vi "iWorx Respiration SubVI.vi"(7 "Waveform Chart":refnum<vi>, 9 "low Threshold":dbl, 10 "high Threshold":dbl) -> (0 "Breath Time History":timestamp[](array[timestamp]), 1 "Instantaneous Breath Rate":dbl format="%.2f", 2 "Avg Breaths per Minute":dbl format="%.2f", 3 "Breath Count":u32)   [LabVIEW 2014]
doc: "This subVI is designed to work with the iWorx Respiration Sensor. It counts the number of times the signal crosses two seperate threasholds. The two threshold method allows it to more accuratly count breaths without noise.s"
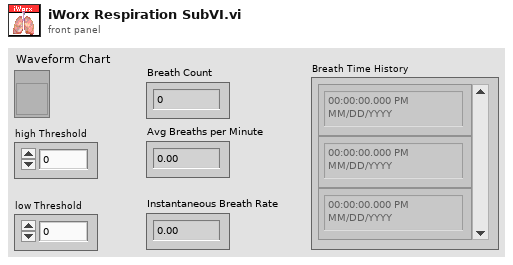
[diagram p1: front panel]
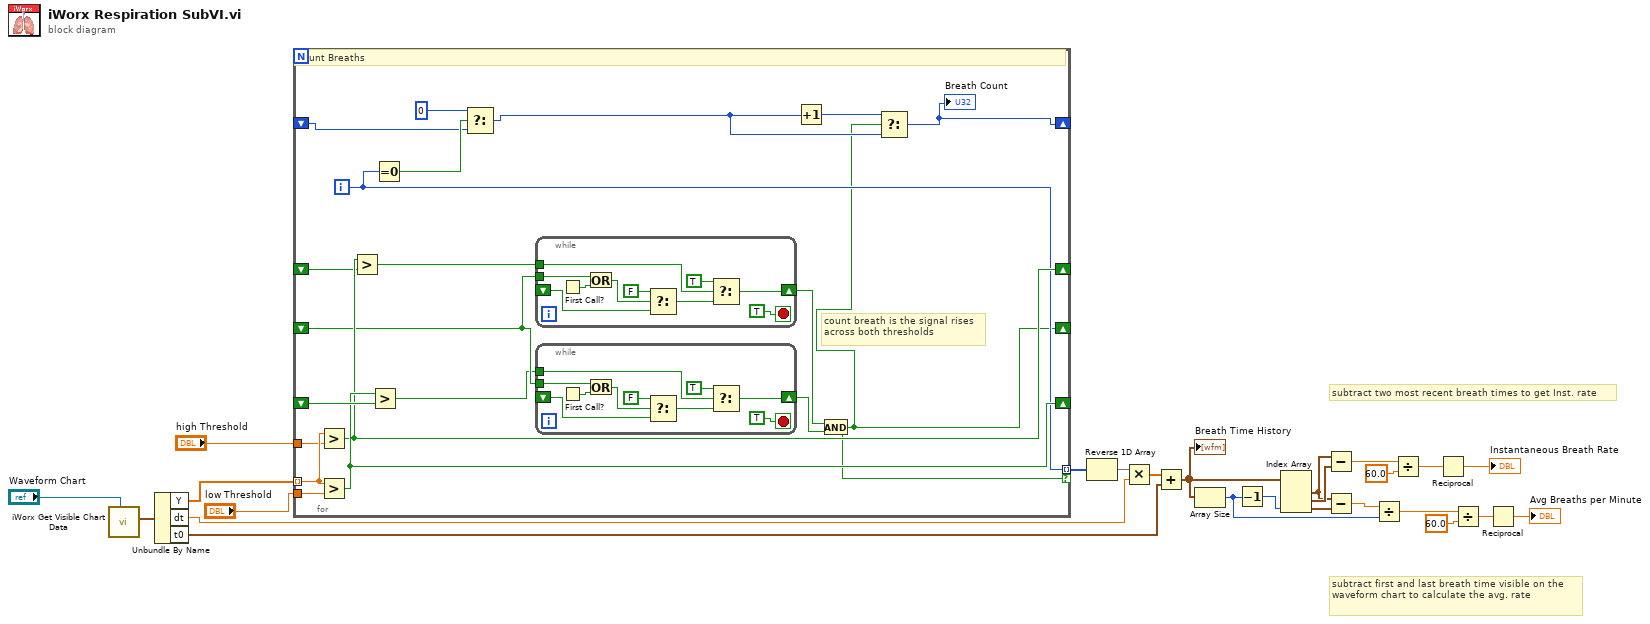
[diagram p0: block diagram]
diagram:
  # "subtract first and last breath time visible on the waveform chart to calculate the avg. rate"
  # "subtract two most recent breath times to get Inst. rate"
  n1 = call "iWorx Get Visible Chart Data.vi"("Selection Chart"="Waveform Chart") -> ("Waveform out"=w24:waveform(dbl))  [unwired: 8 in, 2 out]
  n2 = Unbundle By Name(w24) -> ("Y"=w25:dbl[], "dt"=w16:dbl, "t0"=w7:timestamp)
  n3 = for {
    tunnel: w25 -> [w42] mode=indexing
    shift-right: [w44] -> _
    shift-left: _ -> [w45]
    tunnel: "low Threshold" -> [w43]
    tunnel: "high Threshold" -> [w41]
    shift-right: [w40] -> _
    shift-left: _ -> [w39]
    shift-right: [w28] -> _
    shift-left: _ -> [w37]
    tunnel: [w38] -> w18 mode=indexing if=w28
    shift-right: [w27] -> _
    shift-left: _ -> [w30]
    i -> [w38]
    # "count breath is the signal rises across both thresholds"
    # "Count Breaths"
    n4 = Greater?(x=w42, y=w41) -> (0:w40:bool)
    n5 = Greater?(x=w42, y=w43) -> (0:w44:bool)
    n6 = Greater?(x=w40, y=w39) -> (0:w36:bool)
    n7 = Greater?(x=w44, y=w45) -> (0:w35:bool)
    n8 = Equal To 0?(x=w38) -> (x = 0?=w32:bool)
    n9 = Select(t=u32 0 ("Breath Count"), s=w32, f=w30) -> (s? t:f=w29:u32)
    n10 = while {
      shift-right: [w56] -> w33
      shift-left: _ -> [w59]
      tunnel: w37 -> [w58]
      tunnel: w36 -> [w57]
      stop <- TRUE stop-if-true
      n11 = First Call?() -> (First Call?: T/F=w65:bool)
      n12 = Or(x=w58, y=w65) -> (x .or. y?=w62:bool)
      n13 = Select(t=FALSE, s=w62, f=w59) -> (s? t:f=w61:bool)
      n14 = Select(t=TRUE, s=w57, f=w61) -> (s? t:f=w56:bool)
    }
    n15 = while {
      shift-right: [w46] -> w34
      shift-left: _ -> [w49]
      tunnel: w37 -> [w48]
      tunnel: w35 -> [w47]
      stop <- TRUE stop-if-true
      n16 = First Call?() -> (First Call?: T/F=w55:bool)
      n17 = Or(x=w48, y=w55) -> (x .or. y?=w52:bool)
      n18 = Select(t=FALSE, s=w52, f=w49) -> (s? t:f=w51:bool)
      n19 = Select(t=TRUE, s=w47, f=w51) -> (s? t:f=w46:bool)
    }
    n20 = Increment(x=w29) -> (x+1=w26:u32)
    n21 = And(x=w33, y=w34) -> (x .and. y?=w28:bool)
    n22 = Select(t=w26, s=w28, f=w29) -> (s? t:f=w27:u32)
    "Breath Count" <- w27
  }
  n23 = Reverse 1D Array(array=w18) -> (reversed array=w17:i32[])
  n24 = Multiply(x=w17, y=w16) -> (x*y=w8:dbl[])
  n25 = Add(x=w8, y=w7) -> (x+y=w6:timestamp[])
  "Breath Time History" <- w6
  n26 = Array Size(array=w6) -> (size(s)=w5:i32)
  n27 = Decrement(x=w5) -> (x-1=w12:i32)
  n28 = Index Array(array=w6, index #3=w12) -> (element #1=w11:timestamp, element #2=w15:timestamp, element #3=w10:timestamp)  [unwired: 2 in]
  n29 = Subtract(x=w11, y=w15) -> (x-y=w14:dbl)
  n30 = Subtract(x=w11, y=w10) -> (x-y=w9:dbl)
  n31 = Divide(x=w9, y=w5) -> (x/y=w3:dbl)
  n32 = Divide(x=w14, y=60.0) -> (x/y=w20:dbl)
  n33 = Reciprocal(x=w20) -> (1/x=→"Instantaneous Breath Rate":dbl)
  n34 = Divide(x=w3, y=60.0) -> (x/y=w2:dbl)
  n35 = Reciprocal(x=w2) -> (1/x=→"Avg Breaths per Minute":dbl)
